vi "C Enum To DokuWiki Table.vi"(8 "Error In":errorcluster, 11 "C Enum":string="typedef enum \n    {\n        None                            = 0,\n        Success                         = 1,\n        UDPCacheToSmall                 = 2,\n\n        // Initialization status\n        NetworkNotInitialized           = 10,\n        NetworkInitialized              = 11,\n        DHCPNotBound                    = 12,\n\n        // Epoch status\n        TimeSincePowerUp                = 20,\n        TimeSinceEpoch                  = 21,\n\n        // DNS status\n        DNSIsBusy                       = 30,\n        DNSResolving                    = 31,\n        DNSLookupSuccess                = 32,\n        DNSUninitialized                = 33,\n        DNSResolutionFailed             = 34,\n        DNSHostNameIsNULL               = 35,\n        DNSRecursiveExit                = 36,\n\n        // TCP connect state machine states\n        NotConnected                    = 40,\n        WaitingConnect                  = 41,\n        WaitingReConnect                = 42,\n        Connected                       = 43,\n\n        // other connection status\n        LostConnect                     = 50,\n        ConnectionAlreadyDefined        = 51,\n        SocketError                     = 52,\n        WaitingMACLinkage               = 53,\n        LostMACLinkage                  = 54,\n\n        // write status\n        WriteTimeout                    = 60,\n\n        // read status\n        NoDataToRead                    = 70,\n\n        // Listening status\n        NeedToCallStartListening        = 80,\n        NeedToResumeListening           = 81,\n        AlreadyStarted                  = 82,\n        AlreadyListening                = 83,\n        Listening                       = 84,\n        ExceededMaxPendingAllowed       = 85,\n        MoreCurrentlyPendingThanAllowed = 86,\n        ClientPointerIsNULL             = 87,\n        SocketAlreadyAssignedToClient   = 88,\n        NoPendingClients                = 89,\n        IndexOutOfBounds                = 90,\n\n        // UDP endpoint resolve state machine\n        EndPointNotSet                  = 100,\n\n        // DNSResolving                         \n        ARPResolving                    = 110,\n        AcquiringSocket                 = 111,\n        Finalizing                      = 112,\n        EndPointResolved                = 113,\n\n        // DNSResolutionFailed\n        ARPResolutionFailed             = 120,\n        // SocketError\n \n        // WiFi Stuff below here\n        WFStillScanning                 = 130,\n        WFUnableToGetConnectionID       = 131,\n        WFInvalideConnectionID          = 132,\n        WFAssertHit                     = 133,\n\n    } STATUS;") -> (0 "Error Out":errorcluster, 3 "DokuWiki Table":string="^STATUS^^\r^ Name ^ Value ^\r| None | 0 |\r| Success | 1 |\r| UDPCacheToSmall | 2 |\r| NetworkNotInitialized | 10 |\r| NetworkInitialized | 11 |\r| DHCPNotBound | 12 |\r| TimeSincePowerUp | 20 |\r| TimeSinceEpoch | 21 |\r| DNSIsBusy | 30 |\r| DNSResolving | 31 |\r| DNSLookupSuccess | 32 |\r| DNSUninitialized | 33 |\r| DNSResolutionFailed | 34 |\r| DNSHostNameIsNULL | 35 |\r| DNSRecursiveExit | 36 |\r| NotConnected | 40 |\r| WaitingConnect | 41 |\r| WaitingReConnect | 42 |\r| Connected | 43 |\r| LostConnect | 50 |\r| ConnectionAlreadyDefined | 51 |\r| SocketError | 52 |\r| WaitingMACLinkage | 53 |\r| LostMACLinkage | 54 |\r| WriteTimeout | 60 |\r| NoDataToRead | 70 |\r| NeedToCallStartListening | 80 |\r| NeedToResumeListening | 81 |\r| AlreadyStarted | 82 |\r| AlreadyListening | 83 |\r| Listening | 84 |\r| ExceededMaxPendingAllowed | 85 |\r| MoreCurrentlyPendingThanAllowed | 86 |\r| ClientPointerIsNULL | 87 |\r| SocketAlreadyAssignedToClient | 88 |\r| NoPendingClients | 89 |\r| IndexOutOfBounds | 90 |\r| EndPointNotSet | 100 |\r| ARPResolving | 110 |\r| AcquiringSocket | 111 |\r| Finalizing | 112 |\r| EndPointResolved | 113 |\r| ARPResolutionFailed | 120 |\r| WFStillScanning | 130 |\r| WFUnableToGetConnectionID | 131 |\r| WFInvalideConnectionID | 132 |\r| WFAssertHit | 133 |\r")   [LabVIEW 2011, in "LMH-Toolbox.lvlib" / "LMH-DokuWiki.lvlib"]
uses:
  LMH-DokuWiki.lvlib
panel:
  # "This VI converts a C style Enum into DokuWiki table format.\n(Since the enum size will never be terribly large this VI was written quickly and is not optimized for CPU or memory usage)\n\nInstructions:\n1. Paste a C style enum in the C Enum control below.\n2. Run The VI\n3. Retreive the output from the DokuWiki Table indicator."
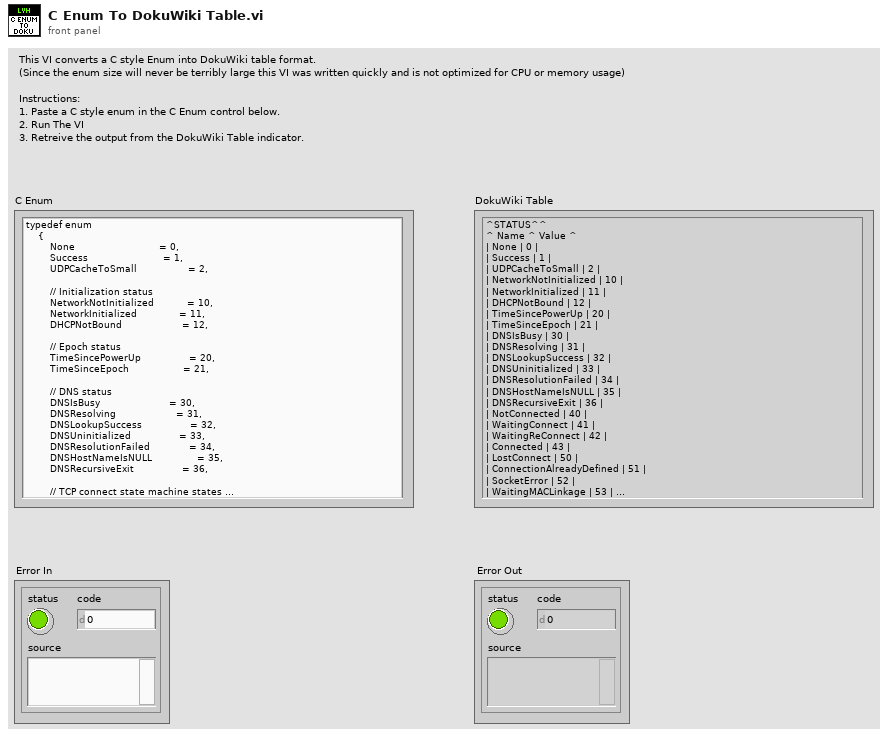
[diagram p1: front panel]
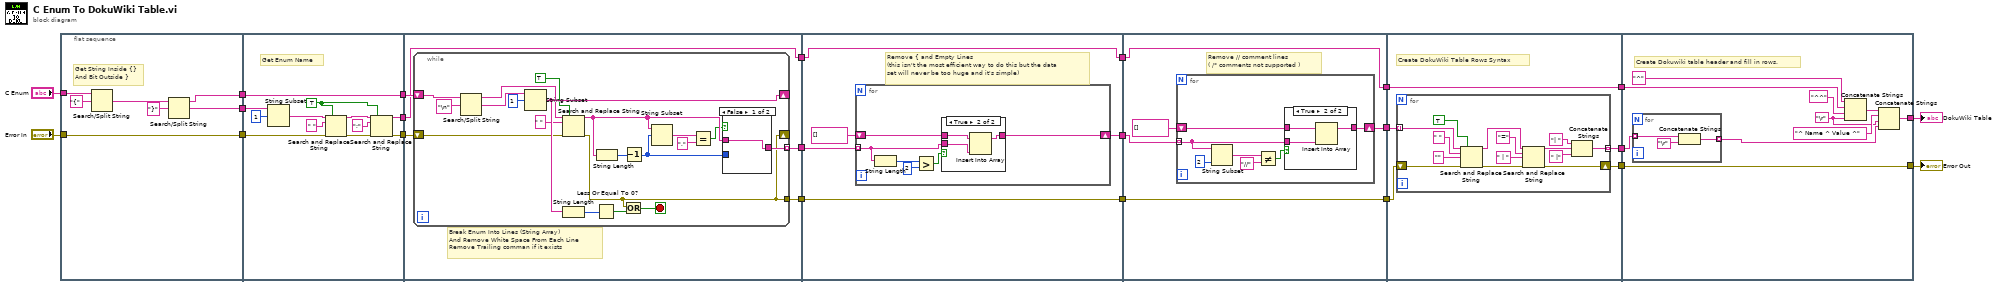
[diagram p0: block diagram]
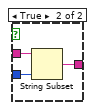
[diagram p2: hidden frame]
diagram:
  n1 = flat-sequence {
    tunnel: "C Enum" -> [w29]
    tunnel: [w25] -> w21
    tunnel: [w24] -> w20
    tunnel: [w23] -> w17
    tunnel: "Error In" -> [w23]
    tunnel: w21 -> [w34]
    tunnel: w20 -> [w41]
    tunnel: [w41] -> w19
    tunnel: [w33] -> w18
    tunnel: w17 -> [w32]
    tunnel: [w31] -> w8
    tunnel: w19 -> [w46]
    tunnel: w18 -> [w45]
    tunnel: [w44] -> w15
    tunnel: [w43] -> w9
    tunnel: w8 -> [w43]
    tunnel: [w42] -> w6
    tunnel: w15 -> [w75]
    tunnel: [w73] -> w14
    tunnel: [w72] -> w10
    tunnel: w9 -> [w72]
    tunnel: w6 -> [w71]
    tunnel: [w71] -> w5
    tunnel: w14 -> [w90]
    tunnel: [w88] -> w13
    tunnel: [w87] -> w11
    tunnel: w10 -> [w87]
    tunnel: w5 -> [w86]
    tunnel: [w86] -> w4
    tunnel: w13 -> [w106]
    tunnel: [w105] -> w12
    tunnel: w11 -> [w104]
    tunnel: [w104] -> w7
    tunnel: w4 -> [w102]
    tunnel: [w103] -> w3
    tunnel: w12 -> [w130]
    tunnel: w7 -> [w129]
    tunnel: [w125] -> w1
    tunnel: w3 -> [w121]
    tunnel: [w121] -> w2
    frame #0 {
      # "Get String Inside {}\nAnd Bit Outside }"
      n2 = Search/Split String(string=w29, search string/char (-)="{") -> (match + rest of string=w27:string)  [unwired: 1 in, 2 out]
      n3 = Search/Split String(string=w27, search string/char (-)="}") -> (substring before match=w24:string, match + rest of string=w25:string)  [unwired: 1 in, 1 out]
    }
    frame #1 {
      w30 = TRUE ("replace all? (F)")
      # "Get Enum Name"
      n4 = String Subset(string=w34, offset (0)=1) -> (substring=w36:string)  [unwired: 1 in]
      n5 = Search and Replace String(replace all?=w30, input string=w36, search string=" ", error in=w32) -> (result string=w38:string, error out=w40:errorcluster)  [unwired: 4 in, 2 out]
      n6 = Search and Replace String(replace all?=w30, input string=w38, search string=";", error in=w40) -> (result string=w31:string, error out=w33:errorcluster)  [unwired: 4 in, 2 out]
    }
    frame #2 {
      # "Break Enum Into Lines (String Array) \nAnd Remove White Space From Each Line\nRemove Trailing comman if it exists"
      n7 = while {
        shift-right: [w61] -> _
        shift-left: w46 -> [w66]
        shift-right: [w47] -> _
        shift-left: w45 -> [w58]
        tunnel: [w50] -> w44 mode=indexing
        tunnel: [w47] -> w42
        stop <- w56 stop-if-true
        # "Break Into Lines"
        n8 = Search/Split String(string=w66, search string/char (-)="\n") -> (substring before match=w60:string, match + rest of string=w63:string)  [unwired: 1 in, 1 out]
        n9 = String Subset(string=w63, offset (0)=1) -> (substring=w61:string)  [unwired: 1 in]
        n10 = Search and Replace String(replace all?=TRUE ("replace all? (F)"), input string=w60, search string=" ", error in=w58) -> (result string=w51:string, error out=w47:errorcluster)  [unwired: 4 in, 2 out]
        n11 = String Length(string=w61) -> (length=w65:i32)
        n12 = Less Or Equal To 0?(x=w65) -> (x <= 0?=w57:bool)
        n13 = String Length(string=w51) -> (length=w54:i32)
        n14 = Or(x=w47, y=w57) -> (x .or. y?=w56:bool)
        n15 = Decrement(x=w54) -> (x-1=w49:i32)
        n16 = String Subset(string=w51, offset (0)=w49) -> (substring=w53:string)  [unwired: 1 in]
        n17 = Equal?(x=w53, y=",") -> (x = y?=w48:bool)
        n18 = case shown="False" w48 {
          tunnel: w51 -> [w67 w70]
          tunnel: [w67 w69] -> w50
          tunnel: w49 -> [_ w68]
          frame False {
          }
          frame True {
            n19 = String Subset(string=w70, length (rest)=w68) -> (substring=w69:string)  [unwired: 1 in]
          }
        }
      }
    }
    frame #3 {
      # "Remove { and Empty Lines\n(this isn't the most efficient way to do this but the data \nset will never be too huge and it's simple)"
      n20 = for {
        tunnel: w75 -> [w77] mode=indexing
        shift-right: [w76] -> w73
        shift-left: string[] [] -> [w81]
        n21 = String Length(string=w77) -> (length=w80:i32)
        n22 = Greater?(x=w80, y=2) -> (0:w78:bool)
        n23 = case shown="True" w78 {
          tunnel: w81 -> [w82 w85]
          tunnel: w77 -> [_ w84]
          tunnel: [w82 w83] -> w76
          frame False {
          }
          frame True {
            n24 = Insert Into Array(array=w85, new element=w84) -> (w83:string[])  [unwired: 1 in]
          }
        }
      }
    }
    frame #4 {
      # "Remove // comment lines\n( /* comments not supported )"
      n25 = for {
        tunnel: w90 -> [w91] mode=indexing
        shift-right: [w92] -> w88
        shift-left: string[] [] -> [w93]
        n26 = String Subset(string=w91, length (rest)=2 ("length (rest)")) -> (substring=w96:string)  [unwired: 1 in]
        n27 = Not Equal?(x=w96, y="//") -> (x != y?=w94:bool)
        n28 = case shown="True" w94 {
          tunnel: w93 -> [w98 w101]
          tunnel: [w98 w100] -> w92
          tunnel: w91 -> [_ w99]
          frame False {
          }
          frame True {
            n29 = Insert Into Array(array=w101, new element=w99) -> (w100:string[])  [unwired: 1 in]
          }
        }
      }
    }
    frame #5 {
      # "Create DokuWiki Table Rows Syntax"
      n30 = for {
        tunnel: [w113] -> w105 mode=indexing
        tunnel: w106 -> [w110] mode=indexing
        shift-right: [w108] -> w103
        shift-left: w102 -> [w107]
        n31 = Search and Replace String(replace all?=TRUE ("replace all? (F)"), input string=w110, search string=" ", replace string="" ("replace string (\"\")"), error in=w107) -> (result string=w118:string, error out=w109:errorcluster)  [unwired: 3 in, 2 out]
        n32 = Search and Replace String(input string=w118, search string="=", replace string=" | " ("replace string (\"\")"), error in=w109) -> (result string=w114:string, error out=w108:errorcluster)  [unwired: 4 in, 2 out]
        n33 = Concatenate Strings("| " ("string"), w114, " |" ("string")) -> (w113:string)
      }
    }
    frame #6 {
      w124 = "\r"
      # "Create Dokuwiki table header and fill in rows."
      n34 = for {
        tunnel: w130 -> [w133] mode=indexing
        tunnel: [w131] -> w123 mode=indexing
        n35 = Concatenate Strings(w133, "\r") -> (w131:string)
      }
      n36 = Concatenate Strings("^" ("string"), w129, "^^" ("string"), w124) -> (w127:string)
      n37 = Concatenate Strings(w127, "^ Name ^ Value ^" ("string"), w124, w123) -> (w125:string)
    }
  }
  "Error Out" <- w2
  "DokuWiki Table" <- w1
